vi "multichannel.lockin.SMO.vi"() -> ()   [LabVIEW 2016]
uses:
  <vilib>/JKI/JKI SMO/SMO/Typedefs/SMOState --Enum.ctl
  SMOs/DAQ/Typedefs/DAQ.Config.ctl
  SMOs/DAQ/Typedefs/PrivateEvents--DAQ.AI.Channels.ctl
  SMOs/DAQ/Typedefs/DAQType.ctl
  SMOs/DAQ/Typedefs/SamplingInfo.ctl
  SMOs/DAQ/Typedefs/SamplingMode.ctl
  SMOs/DAQmx.AI/Typedefs/DAQmx.AI.Config.ctl
  SMOs/DAQmx.AO/Typedefs/DAQmx.AO.Config.ctl
  SMOs/DAQmx/DAQmx.lvclass
  C:/user/patrick/hg/lockin.SMO/lvsrc/SMOs/DAQ/DAQ.lvclass
  SMOs/DAQmx.AI/DAQmx.AI.lvclass
  C:/user/patrick/hg/lockin.SMO/lvsrc/SMOs/DAQmx/DAQmx.lvclass
  SMOs/DAQmx.AO/DAQmx.AO.lvclass
  SMOs/DAQ/DAQ.lvclass
  C:/Program Files (x86)/National Instruments/LabVIEW 2016/vi.lib/JKI/JKI SMO/SMO/SMO.lvclass
  <vilib>/JKI/JKI SMO/SMO/SMO.lvclass
panel:
  in  "DAQ.Config (AO)":T1={"Channels"="", "DAQType"=enum."AO", "minimum value"=-5.0, "maximum value"=5.0, "sampling info"={"Fs"=1000.0, "#s"=1000.0}, "SamplingMode"=enum."Continuous"} {"maximum value" format="%0.2f"; "minimum value" format="%0.2f"}
  in  "DAQmx Physical Channels (AO)":tag="PXI1Slot2/ao0:1, PXI1Slot3/ao0:1, PXI1Slot4/ao0:1, PXI1Slot5/ao0:1"
  in  "DAQmx.AO.config":T6={"output terminal configuration"=-1} {"output terminal configuration" items=["Default"=-1, "RSE"=10083, "Differential"=10106, "Pseudodifferential"=12529]}
  in  "DAQmx.AI.config":T7={"AI.Coupling"=10045, "input terminal configuration "=-1} {"input terminal configuration" items=["default"=-1, "RSE"=10083, "NRSE"=10078, "Differential"=10106, "Pseudodifferential"=12529]; "AI.Coupling" items=["AC"=10045, "DC"=10050, "GND"=10066]}
  in  "DAQmx Physical Channels (AI)":tag="PXI1Slot2/ai0:1, PXI1Slot3/ai0:1, PXI1Slot4/ai0:1, PXI1Slot5/ai0:1"
  in  "DAQ.Config (AI)":T1={"Channels"="", "DAQType"=enum."AI", "minimum value"=-5.0, "maximum value"=5.0, "sampling info"={"Fs"=1000.0, "#s"=1000.0}, "SamplingMode"=enum."Continuous"} {"maximum value" format="%0.2f"; "minimum value" format="%0.2f"}
  in  "Simulate?":bool
  out "Write":waveform(dbl)[](graph)
  out "Read":T8(graph)
  out "SMO State":T9
  out "error out":errorcluster
  in  "Stop":bool
  # "Multichannel Lockin SMO Test Launcher"
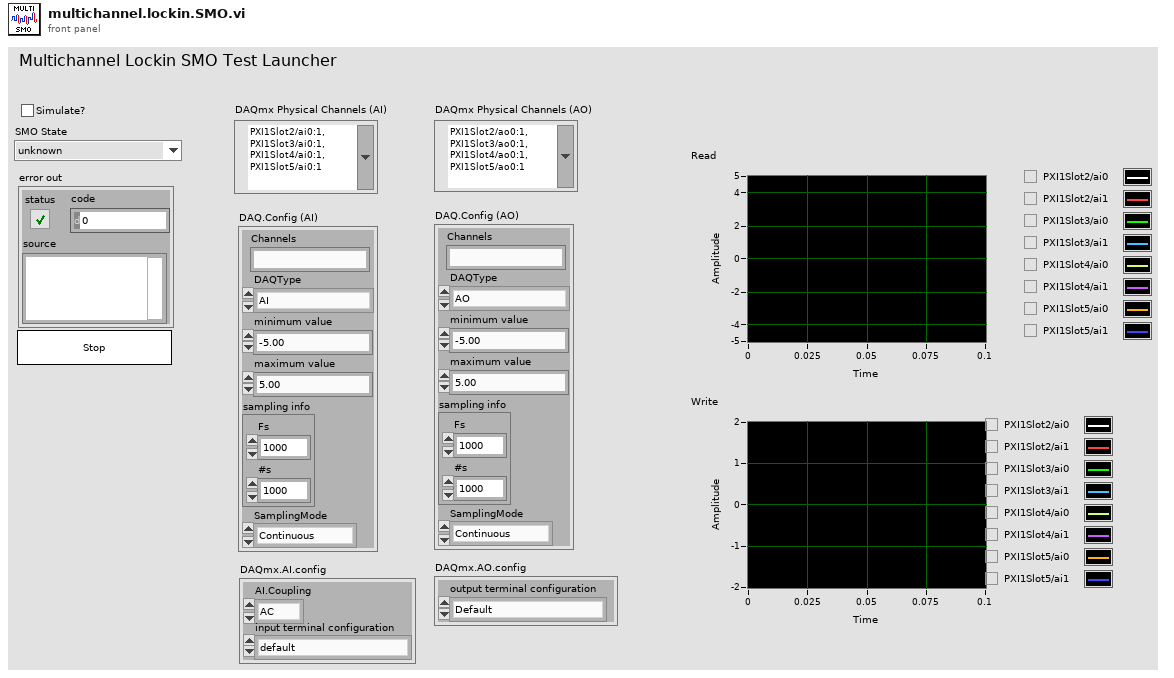
[diagram p1: front panel]
types:
  T1 = typedef "DAQ.lvclass/DAQ.Config.ctl" = cluster{"Channels":T2, "DAQType":T3, "minimum value":dbl, "maximum value":dbl, "sampling info":T4, "SamplingMode":T5}
  T2 = typedef "PrivateEvents--DAQ.AI.Channels.ctl" = string
  T3 = typedef "DAQ.lvclass/DAQType.ctl" = enum16{"AI", "AO"}
  T4 = typedef "DAQ.lvclass/SamplingInfo.ctl" = cluster{"Fs":dbl, "#s":dbl}
  T5 = typedef "DAQ.lvclass/SamplingMode.ctl" = enum16{"Continuous", "Finite"}
  T6 = typedef "DAQmx.AO.lvclass/DAQmx.AO.Config.ctl" = cluster{"output terminal configuration":i32}
  T7 = typedef "DAQmx.AI.lvclass/DAQmx.AI.Config.ctl" = cluster{"AI.Coupling":i32, "input terminal configuration ":i32}
  T8 = typedef "DAQ.lvclass/PublicEvents--DAQ.Read.ctl" = waveform(dbl)[]
  T9 = typedef "SMO.lvclass/SMOState --Enum.ctl" = enum16{"unknown", "Created", "Started", "Stopped"}
  T10 = typedef "SMO.lvclass/Public Events.ctl" = cluster{"Error":refnum<user-event>, "State":refnum<user-event>, "Reserve State":refnum<user-event>}
  T11 = typedef "DAQ.lvclass/PublicEvents--Cluster.ctl" = cluster{"Read":refnum<user-event>, "Write":refnum<user-event>}
  T12 = typedef "DAQ.lvclass/PublicEvents--DAQ.Write.ctl" = waveform(dbl)[]
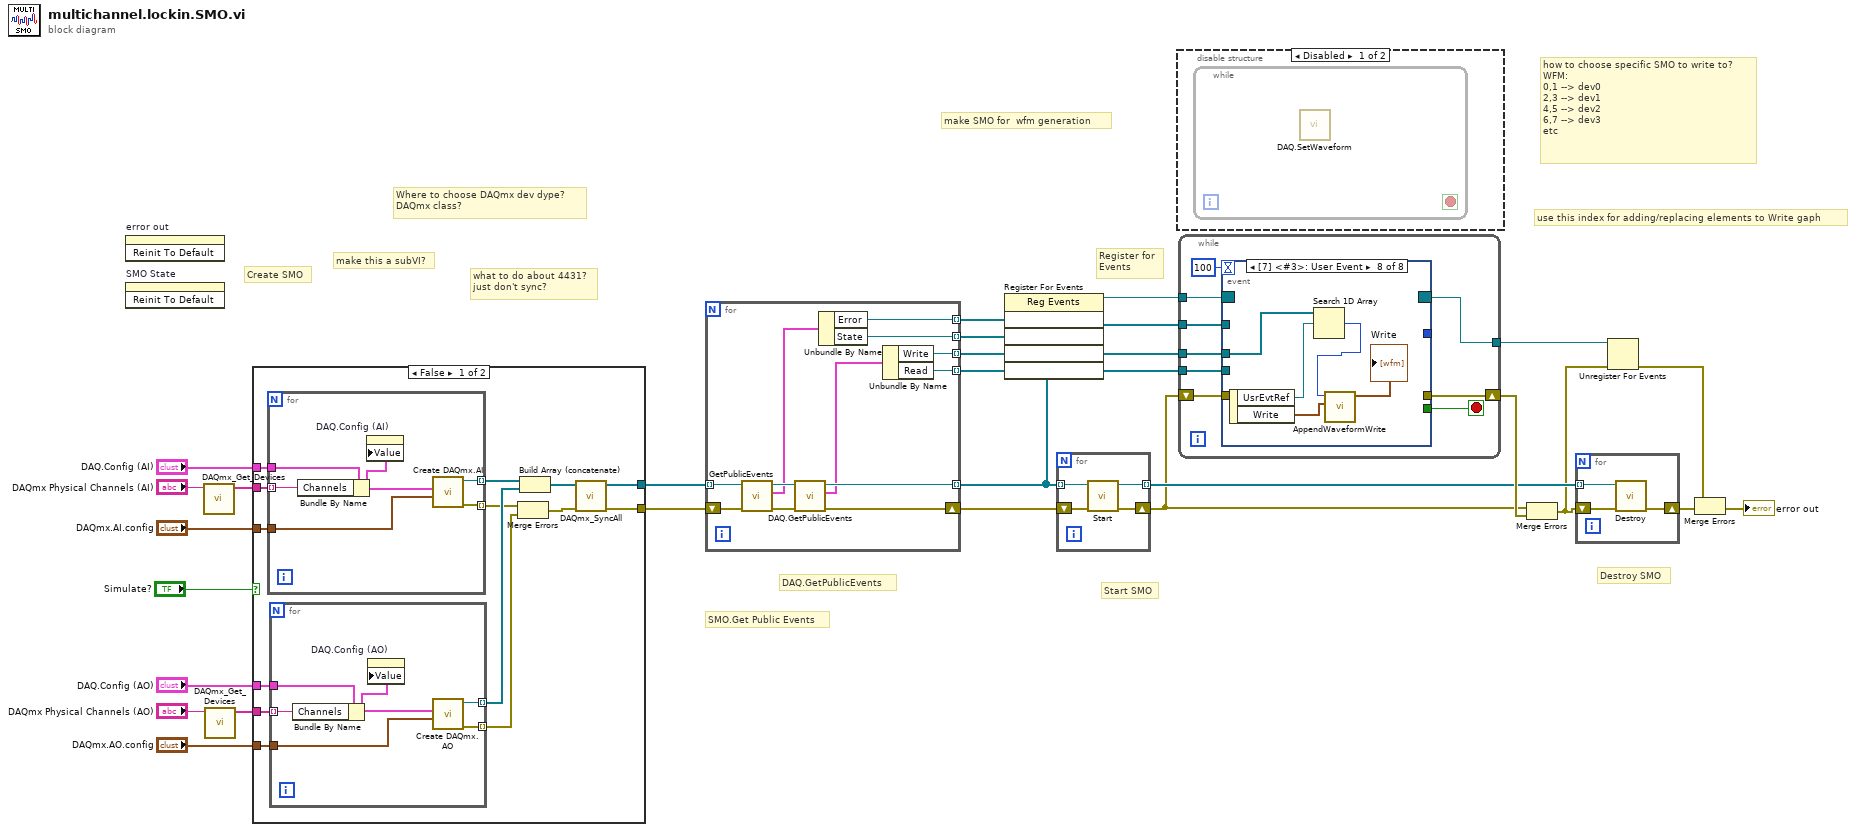
[diagram p0: block diagram]
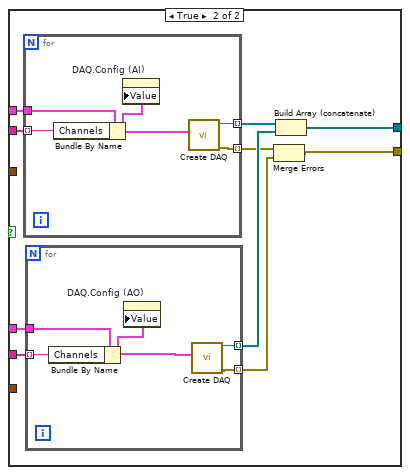
[diagram p3: hidden frame]
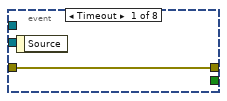
[diagram p4: hidden frame]
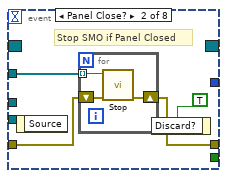
[diagram p5: hidden frame]
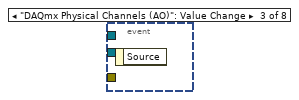
[diagram p6: hidden frame]
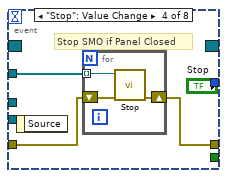
[diagram p7: hidden frame]
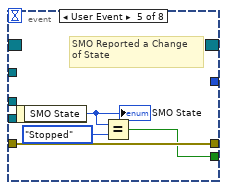
[diagram p8: hidden frame]
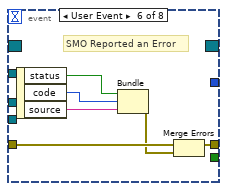
[diagram p9: hidden frame]
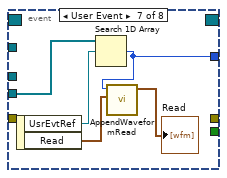
[diagram p10: hidden frame]
diagram:
  # "Where to choose DAQmx dev dype?\nDAQmx class?"
  # "what to do about 4431?\njust don't sync?"
  # "make this a subVI?"
  # "how to choose specific SMO to write to?\nWFM:\n0,1 --> dev0\n2,3 --> dev1\n4,5 --> dev2\n6,7 --> dev3\netc"
  # "use this index for adding/replacing elements to Write gaph"
  # "make SMO for  wfm generation"
  # "DAQ.GetPublicEvents"
  # "SMO.Get Public Events"
  # "Start SMO"
  # "Destroy SMO"
  # "Create SMO"
  # "Register for Events"
  n1 = invoke on="error out" class="Clust (strict)" method="Reinit To Default"() -> ()  [unwired: 3 in, 3 out]
  n2 = invoke on="SMO State" class="Enum (strict)" method="Reinit To Default"() -> ()  [unwired: 3 in, 3 out]
  n3 = call "DAQmx_Get_Devices.vi"("DAQmx Physical Channel"="DAQmx Physical Channels (AI)") -> ("Channels Array"=w15:string[])  [unwired: 10 in]
  n4 = call "DAQmx_Get_Devices.vi"("DAQmx Physical Channel"="DAQmx Physical Channels (AO)") -> ("Channels Array"=w12:string[])  [unwired: 10 in]
  n5 = case shown="False" "Simulate?" {
    tunnel: "DAQ.Config (AO)" -> [w40 w62]
    tunnel: "DAQmx.AO.config" -> [w39 _]
    tunnel: w15 -> [w38 w61]
    tunnel: "DAQ.Config (AI)" -> [w37 w60]
    tunnel: "DAQmx.AI.config" -> [w36 _]
    tunnel: w12 -> [w35 w59]
    tunnel: [w30 w53] -> w10
    tunnel: [w29 w54] -> w9
    frame False {
      n6 = for {
        tunnel: w38 -> [w52] mode=indexing
        tunnel: w37 -> [w51]
        tunnel: w36 -> [w49]
        tunnel: [w48] -> w32 mode=indexing
        tunnel: [w47] -> w34 mode=indexing
        n7 = Bundle By Name(cluster=w51, "Channels"=w52) -> (w50:T1)
        n8 = property on="DAQ.Config (AI)" class="Clust (strict)"("Value"=w50) -> ()  [unwired: 2 in, 2 out]
        n9 = call "Create DAQmx.AI.vi"("DAQmx.AI.config"=w49, "DAQ.config"=w50) -> ("error out"=w48:errorcluster, "DAQmx.AI out"=w47:refnum<class "DAQmx.AI.lvclass">)  [unwired: 8 in]
      }
      n10 = for {
        tunnel: w40 -> [w46]
        tunnel: w39 -> [w43]
        tunnel: w35 -> [w44] mode=indexing
        tunnel: [w42] -> w33 mode=indexing
        tunnel: [w41] -> w31 mode=indexing
        n11 = Bundle By Name(cluster=w46, "Channels"=w44) -> (w45:T1)
        n12 = property on="DAQ.Config (AO)" class="Clust (strict)"("Value"=w45) -> ()  [unwired: 2 in, 2 out]
        n13 = call "Create DAQmx.AO.vi"("DAQmx.AO.config"=w43, "DAQ.Config"=w45) -> ("error out"=w41:errorcluster, "DAQmx.AO out"=w42:refnum<class "DAQmx.AO.lvclass">)  [unwired: 8 in]
      }
      n14 = Merge Errors(w32, w31) -> (w27:errorcluster)
      n15 = Build Array (concatenate)(w34, w33) -> (w28:refnum<class "DAQmx.lvclass">[])
      n16 = call "DAQmx_SyncAll.vi"("error in (no error)"=w27, "Array in"=w28) -> ("error out"=w30:errorcluster, "Array out"=w29:refnum<class "DAQmx.lvclass">[])  [unwired: 8 in]
    }
    frame True {
      n17 = for {
        tunnel: w61 -> [w72] mode=indexing
        tunnel: w60 -> [w71]
        tunnel: [w68] -> w56 mode=indexing
        tunnel: [w69] -> w58 mode=indexing
        n18 = Bundle By Name(cluster=w71, "Channels"=w72) -> (w70:T1)
        n19 = property on="DAQ.Config (AI)" class="Clust (strict)"("Value"=w70) -> ()  [unwired: 2 in, 2 out]
        n20 = call "Create DAQ.vi"("DAQ.Config"=w70) -> ("error out"=w68:errorcluster, "DAQ out"=w69:refnum<class "DAQ.lvclass">)  [unwired: 9 in]
      }
      n21 = for {
        tunnel: w62 -> [w67]
        tunnel: w59 -> [w66] mode=indexing
        tunnel: [w65] -> w57 mode=indexing
        tunnel: [w64] -> w55 mode=indexing
        n22 = Bundle By Name(cluster=w67, "Channels"=w66) -> (w63:T1)
        n23 = property on="DAQ.Config (AO)" class="Clust (strict)"("Value"=w63) -> ()  [unwired: 2 in, 2 out]
        n24 = call "Create DAQ.vi"("DAQ.Config"=w63) -> ("error out"=w64:errorcluster, "DAQ out"=w65:refnum<class "DAQ.lvclass">)  [unwired: 9 in]
      }
      n25 = Merge Errors(w56, w55) -> (w53:errorcluster)
      n26 = Build Array (concatenate)(w58, w57) -> (w54:refnum<class "DAQ.lvclass">[])
    }
  }
  n27 = for {
    tunnel: [w83] -> w11 mode=indexing
    tunnel: w9 -> [w82] mode=indexing
    shift-right: [w79] -> w20
    shift-left: w10 -> [w81]
    tunnel: [w78] -> w2 mode=indexing
    tunnel: [w76] -> w1 mode=indexing
    tunnel: [w74] -> w6 mode=indexing
    tunnel: [w73] -> w5 mode=indexing
    n28 = call <vilib>:"GetPublicEvents.vi"("error in (no error)"=w81, "SMO"=w82) -> ("error out"=w84:errorcluster, "Public Events"=w75:T10, "SMO out"=w80:refnum<class "DAQ.lvclass">)  [unwired: 7 in]
    n29 = call "DAQ.GetPublicEvents.vi"("error in (no error)"=w84, "DAQ"=w80) -> ("error out"=w79:errorcluster, "Public Events"=w77:T11, "DAQ out"=w83:refnum<class "DAQ.lvclass">)  [unwired: 7 in]
    n30 = Unbundle By Name(w75) -> ("Error"=w73:refnum<user-event>, "State"=w74:refnum<user-event>)
    n31 = Unbundle By Name(w77) -> ("Write"=w78:refnum<user-event>, "Read"=w76:refnum<user-event>)
  }
  n32 = register-events(w5, w6, w2, w1) -> (reference out=w4:refnum<event-registration>)  [unwired: 2 in, 1 out]
  n33 = for {
    shift-right: [w87] -> w21
    shift-left: w20 -> [w85]
    tunnel: w11 -> [w86] mode=indexing
    tunnel: [w88] -> w22 mode=indexing
    n34 = call <vilib>:"Start.vi"("error in (no error)"=w85, "SMO"=w86) -> ("error out"=w87:errorcluster, "SMO out"=w88:refnum<class "DAQ.lvclass">)  [unwired: 8 in]
  }
  n35 = disable-structure shown="Disabled" {
    frame Disabled {
      n36 = while {
        stop <- _ stop-if-true
        n37 = call "DAQ.SetWaveform.vi"() -> ()  [unwired: 10 in, 2 out]
      }
    }
    frame Enabled {
    }
  }
  n38 = while {
    shift-right: [w96] -> w26
    shift-left: w21 -> [w95]
    tunnel: w4 -> [w94]
    tunnel: [w93] -> w3
    tunnel: w11 -> [w91]
    tunnel: w2 -> [w90]
    tunnel: w1 -> [w89]
    stop <- w97 stop-if-true
    n39 = event shown="[7] <#3>: User Event" {
      selector: w94 -> [_ _ _ _ _ _ _ _]
      dyn-events: [_ _ _ _ _ _ _ _] -> w93
      timeout: 100 -> [_ _ _ _ _ _ _ _]
      tunnel: [_ _ _ _ w112 _ _ _] -> w97
      tunnel: [w98 w102 _ w108 w115 w119 _ _] -> w96
      tunnel: w95 -> [w98 w99 _ w107 w115 w117 _ _]
      tunnel: w91 -> [_ w100 _ w106 _ _ _ _]
      tunnel: w90 -> [_ _ _ _ _ _ _ w131]
      tunnel: w89 -> [_ _ _ _ _ _ w126 _]
      tunnel: [_ _ _ _ _ _ w122 _] -> _
      event Timeout {
        n40 = event-data() -> ()  [unwired: 1 in, 1 out]
      }
      event Panel Close? {
        # "Stop SMO if Panel Closed"
        n41 = event-data() -> ()  [unwired: 1 in, 1 out]
        n42 = for {
          shift-right: [w105] -> w102
          shift-left: w99 -> [w104]
          tunnel: w100 -> [w103] mode=indexing
          n43 = call <vilib>:"Stop.vi"("error in (no error)"=w104, "SMO"=w103) -> ("error out"=w105:errorcluster)  [unwired: 8 in, 1 out]
        }
        n44 = event-data("Discard?"=TRUE ("OK")) -> ()  [unwired: 1 in, 1 out]
      }
      event "DAQmx Physical Channels (AO)": Value Change {
        n45 = event-data() -> ()  [unwired: 1 in, 1 out]
      }
      event "Stop": Value Change {
        # "Stop SMO if Panel Closed"
        n46 = event-data() -> ()  [unwired: 1 in, 1 out]
        n47 = for {
          shift-right: [w111] -> w108
          shift-left: w107 -> [w110]
          tunnel: w106 -> [w109] mode=indexing
          n48 = call <vilib>:"Stop.vi"("error in (no error)"=w110, "SMO"=w109) -> ("error out"=w111:errorcluster)  [unwired: 8 in, 1 out]
        }
      }
      event User Event {
        # "SMO Reported a Change\nof State"
        n49 = event-data() -> ("SMO State"=w114:T9)  [unwired: 1 in]
        "SMO State" <- w114
        n50 = Equal?(x=w114, y=SMOState_--Enum."Stopped") -> (x = y?=w112:bool)
      }
      event User Event {
        # "SMO Reported an Error"
        n51 = event-data() -> ("status"=w118:bool, "code"=w121:i32, "source"=w120:string)  [unwired: 1 in]
        n52 = Bundle("status"=w118, "code"=w121, "source"=w120) -> (w116:errorcluster)  [unwired: 1 in]
        n53 = Merge Errors(w117, w116) -> (w119:errorcluster)
      }
      event User Event {
        n54 = event-data() -> ("UsrEvtRef"=w125:refnum<user-event>, "Read"=w124:T8)  [unwired: 1 in]
        n55 = Search 1D Array(1D array=w126, element=w125) -> (index of element=w122:i32)  [unwired: 1 in]
        n56 = call "AppendWaveformRead.vi"("WFM in"=w124, "index of element"=w122) -> ("WFM out"=→"Read":T8)  [unwired: 9 in]
      }
      event User Event {
        n57 = event-data() -> ("UsrEvtRef"=w130:refnum<user-event>, "Write"=w129:T12)  [unwired: 1 in]
        n58 = Search 1D Array(1D array=w131, element=w130) -> (index of element=w128:i32)  [unwired: 1 in]
        n59 = call "AppendWaveformWrite.vi"("WFM in in"=w129, "index of element"=w128) -> ("WFM out"=→"Write":T12)  [unwired: 9 in]
      }
    }
  }
  n60 = Merge Errors(w21, w26) -> (w7:errorcluster)
  n61 = for {
    tunnel: w22 -> [w132] mode=indexing
    shift-right: [w134] -> w23
    shift-left: w7 -> [w133]
    n62 = call <vilib>:"Destroy.vi"("error in (no error)"=w133, "SMO"=w132) -> ("error out"=w134:errorcluster)  [unwired: 9 in]
  }
  n63 = Unregister For Events(event registration refnum=w3, error in=w7) -> (error out=w25:errorcluster)
  n64 = Merge Errors(w25, w23) -> (→"error out":errorcluster)
